vi "Write Outputs False.vi"(8 "error in (no error)":errorcluster, 11 "Digital Writer in":refnum<class "Digital Writer.lvclass">) -> (0 "error out":errorcluster, 3 "Digital Writer out":refnum<class "Digital Writer.lvclass">)   [LabVIEW 2024, in "DAQmx Actor.lvlib" / "Digital Writer.lvclass"]
uses:
  Digital Writer.lvclass
  Digital Writer.lvclass/Digital Writer.ctl
  <resource>/objmgr/daqmx.rc
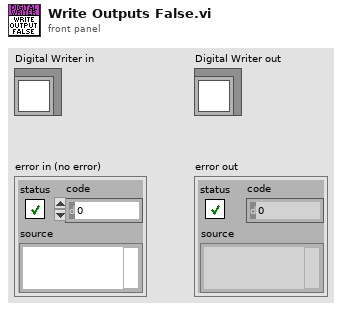
[diagram p1: front panel]
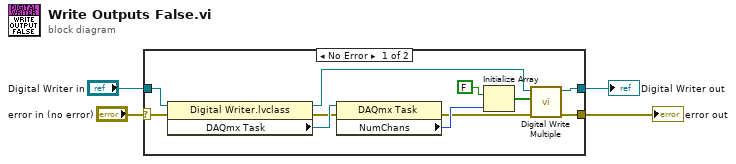
[diagram p0: block diagram]
diagram:
  n1 = case shown="No Error" "error in (no error)" {
    selector: "error in (no error)" -> [w10 w17]
    tunnel: [w6 w17] -> w3
    tunnel: [w7 w16] -> w1
    tunnel: "Digital Writer in" -> [w15 w16]
    frame No Error {
      n2 = property class="Digital Writer.lvclass"(reference=w15, error in=w10) -> (reference out=w8:refnum<class "Digital Writer.lvclass">, error out=w11:errorcluster, "DAQmx Task"=w14:refnum<k21>)
      n3 = property class="DAQmx Task"(reference=w14, error in=w11) -> (error out=w5:errorcluster, "NumChans"=w12:u32)  [unwired: 1 out]
      n4 = Initialize Array(FALSE, w12) -> (w9:bool[])
      n5 = call-dynamic "Digital Write Multiple.vi"("error in (no error)"=w5, "Digital Data"=w9, "Digital Writer in"=w8) -> ("error out"=w6:errorcluster, "Digital Writer out"=w7:refnum<class "Digital Writer.lvclass">)  [unwired: 7 in]
    }
    frame Error {
    }
  }
  "error out" <- w3
  "Digital Writer out" <- w1
